vi "get_target_XYZ_pos.vi"(8 "error in (no error)":errorcluster caption="错误输入（无错误）", 11 "MotorSystem 输入":refnum<class "MotorSystem.lvclass">) -> (0 "error out":errorcluster caption="错误输出", 2 "target":cluster{"X":dbl, "Y":dbl, "Z":dbl}={"X"=0.0, "Y"=0.0, "Z"=200.0}, 3 "MotorSystem 输出":refnum<class "MotorSystem.lvclass">)   [LabVIEW 2016, in "MotionControl_UFO_3DOF.lvlib" / "MotorSystem.lvclass"]
uses:
  <userlib>/MotionControl_UFO_3DOF/MotorSystem/MotorSystem.lvclass
  <userlib>/MotionControl_UFO_3DOF/MotorSystem/MotorSystem.lvclass/MotorSystem.ctl
  <userlib>/MotionControl_UFO_3DOF/OneMotion/OneMotion.lvclass/OneMotion.ctl
  <userlib>/MotionControl_UFO_3DOF/OneMotion/OneMotion.lvclass
panel:
  in  "target pos with offset":cluster{"X":dbl, "Y":dbl, "Z":dbl}={"X"=0.0, "Y"=0.0, "Z"=200.0}
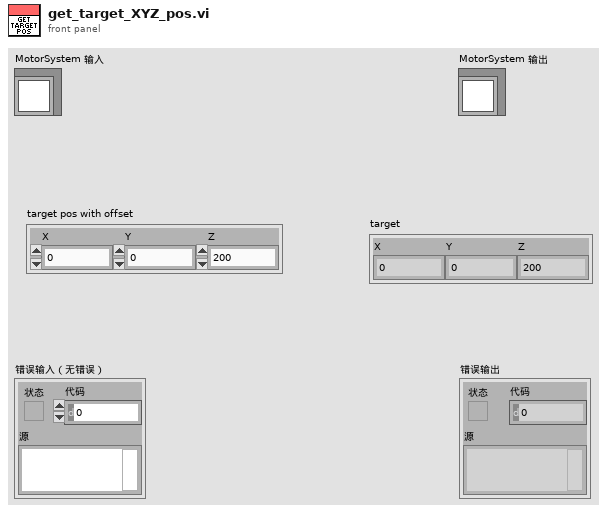
[diagram p1: front panel]
types:
  T1 = typedef "MotionControl_UFO_3DOF.lvlib/MotorSystem.lvclass/MotionCluster.ctl" = cluster{"OneMotion.lvclass":refnum<class "OneMotion.lvclass">, "connected?":bool, "default enabled?":bool, "enabled?":bool}
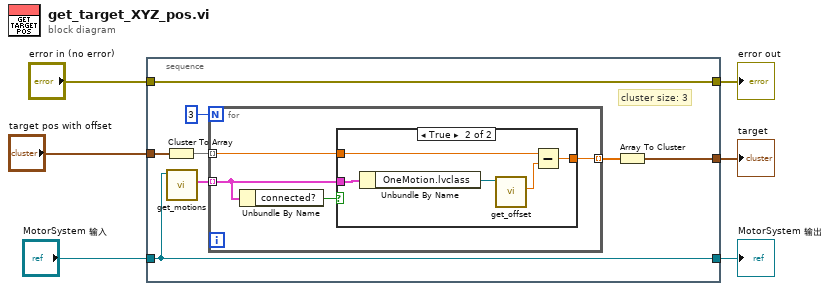
[diagram p0: block diagram]
diagram:
  n1 = stacked-sequence {
    tunnel: [w14] -> w6
    tunnel: [w13] -> w4
    tunnel: "MotorSystem 输入" -> [w13]
    tunnel: "error in (no error)" -> [w14]
    tunnel: "target pos with offset" -> [w8]
    tunnel: [w9] -> w2
    frame #0 {
      # "cluster size: 3"
      n2 = Cluster To Array(cluster=w8) -> (array=w7:dbl[])
      n3 = call <userlib>:"get_motions.vi"("MotorSystem输入"=w13) -> ("motions"=w12:T1[])  [unwired: 8 in, 2 out]
      n4 = for {
        N: 3 -> [_]
        tunnel: w12 -> [w16] mode=indexing
        tunnel: w7 -> [w18] mode=indexing
        tunnel: [w17] -> w10 mode=indexing
        n5 = Unbundle By Name(w16) -> ("connected?"=w15:bool)
        n6 = case shown="True" w15 {
          tunnel: w18 -> [_ w21]
          tunnel: [_ w20] -> w17
          tunnel: w16 -> [_ w19]
          frame False {
          }
          frame True {
            n7 = Unbundle By Name(w19) -> ("OneMotion.lvclass"=w23:refnum<class "OneMotion.lvclass">)
            n8 = call <userlib>:"get_offset.vi"("OneMotion输入"=w23) -> ("offset"=w22:dbl)  [unwired: 8 in, 2 out]
            n9 = Subtract(x=w21, y=w22) -> (x-y=w20:dbl)
          }
        }
      }
      n10 = Array To Cluster(array=w10) -> (cluster=w9:cluster{"[0]":dbl, "[1]":dbl, "[2]":dbl})
    }
  }
  "error out" <- w6
  "MotorSystem 输出" <- w4
  "target" <- w2
